vi "readROIXML.vi"(8 "error in (no error)":errorcluster, 11 "ImageStreamViewer in":refnum<class "ImageStreamViewer.lvclass">) -> (0 "error out":errorcluster, 3 "ImageStreamViewer out":refnum<class "ImageStreamViewer.lvclass">)   [LabVIEW 2009, in "Views.lvlib" / "Camera.lvlib" / "ImageStreamViewer.lvclass"]
uses:
  ImageStreamViewer.lvclass
  ImageStreamViewer.lvclass/ImageStreamViewer.ctl
  Tools/NativeXML/NativeXML.lvclass
  Tools/Filing/FileSystem/FileSystem.lvclass
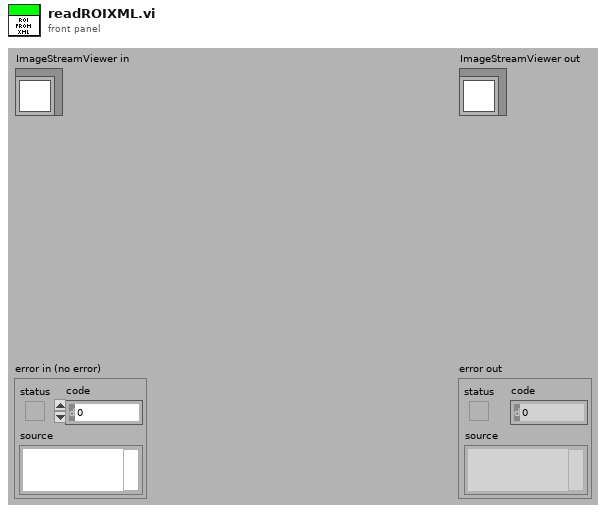
[diagram p1: front panel]
types:
  T1 = cluster{"Left":i32, "Top":i32, "Right":i32, "Bottom":i32}
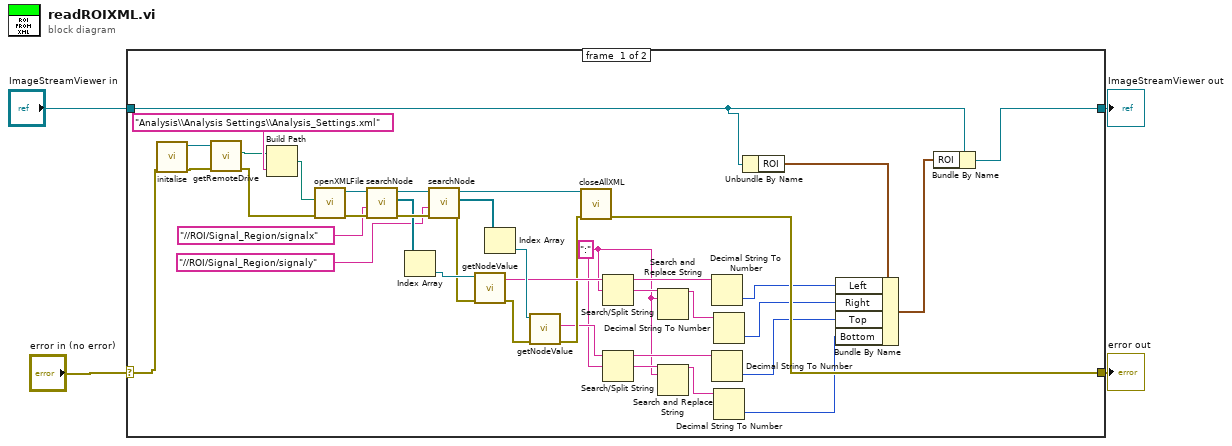
[diagram p0: block diagram]
diagram:
  n1 = case shown="No Error" "error in (no error)" {
    selector: "error in (no error)" -> [w26 w45]
    tunnel: [w25 w45] -> w3
    tunnel: [w8 w44] -> w1
    tunnel: "ImageStreamViewer in" -> [w9 w44]
    frame #0 {
      w7 = ":"
      n2 = call "initalise.vi"("error in (no error)"=w26) -> ("error out"=w32:errorcluster, "FileSystem out"=w31:refnum<class "FileSystem.lvclass">)  [unwired: 9 in]
      n3 = call "getRemoteDrive.vi"("error in (no error)"=w32, "FileSystem in"=w31) -> ("error out"=w27:errorcluster, "RemoteDrive"=w29:path)  [unwired: 7 in, 1 out]
      n4 = Build Path(base path=w29, name or relative path="Analysis\\Analysis Settings\\Analysis_Settings.xml") -> (appended path=w28:path)
      n5 = call "openXMLFile.vi"("error in (no error)"=w27, "Path"=w28) -> ("error out"=w42:errorcluster, "NativeXML out"=w43:refnum<class "NativeXML.lvclass">)  [unwired: 8 in]
      n6 = call "searchNode.vi"("error in (no error)"=w42, "searchXPath"="//ROI/Signal_Region/signalx", "NativeXML in"=w43) -> ("error out"=w40:errorcluster, "nodeArray"=w39:refnum<class "NativeXML.lvclass">[], "NativeXML out"=w41:refnum<class "NativeXML.lvclass">)  [unwired: 6 in]
      n7 = Index Array(array=w39) -> (element=w38:refnum<class "NativeXML.lvclass">)  [unwired: 1 in]
      n8 = call "searchNode.vi"("error in (no error)"=w40, "searchXPath"="//ROI/Signal_Region/signaly", "NativeXML in"=w41) -> ("error out"=w34:errorcluster, "nodeArray"=w37:refnum<class "NativeXML.lvclass">[], "NativeXML out"=w33:refnum<class "NativeXML.lvclass">)  [unwired: 6 in]
      n9 = call "getNodeValue.vi"("error in (no error)"=w34, "NativeXML in"=w38) -> ("error out"=w35:errorcluster, "Value"=w24:string)  [unwired: 7 in, 1 out]
      n10 = Index Array(array=w37) -> (element=w36:refnum<class "NativeXML.lvclass">)  [unwired: 1 in]
      n11 = call "getNodeValue.vi"("error in (no error)"=w35, "NativeXML in"=w36) -> ("error out"=w20:errorcluster, "Value"=w16:string)  [unwired: 7 in, 1 out]
      n12 = call "closeAllXML.vi"("error in (no error)"=w20, "NativeXML in"=w33) -> ("error out"=w25:errorcluster)  [unwired: 9 in]
      n13 = Search/Split String(string=w24, search string/char (-)=w7) -> (substring before match=w22:string, match + rest of string=w23:string)  [unwired: 1 in, 1 out]
      n14 = Search/Split String(string=w16, search string/char (-)=w7) -> (substring before match=w18:string, match + rest of string=w19:string)  [unwired: 1 in, 1 out]
      n15 = Search and Replace String(input string=w23, search string=w7) -> (result string=w21:string)  [unwired: 6 in, 3 out]
      n16 = Search and Replace String(input string=w19, search string=w7) -> (result string=w17:string)  [unwired: 6 in, 3 out]
      n17 = Decimal String To Number(string=w22) -> (number=w13:i32)  [unwired: 2 in, 1 out]
      n18 = Decimal String To Number(string=w18) -> (number=w12:i32)  [unwired: 2 in, 1 out]
      n19 = Decimal String To Number(string=w21) -> (number=w14:i32)  [unwired: 2 in, 1 out]
      n20 = Decimal String To Number(string=w17) -> (number=w11:i32)  [unwired: 2 in, 1 out]
      n21 = Unbundle By Name(w9) -> ("ROI"=w15:T1)
      n22 = Bundle By Name(cluster=w15, "Left"=w13, "Right"=w14, "Top"=w12, "Bottom"=w11) -> (w10:T1)
      n23 = Bundle By Name(cluster=w9, "ROI"=w10) -> (w8:refnum<class "ImageStreamViewer.lvclass">)
    }
    frame #1 {
    }
  }
  "error out" <- w3
  "ImageStreamViewer out" <- w1
